vi "Desvio padrão normatizado.vi"(1 "Dados out":T1) -> (0 "Desvios das deformações":dbl[](array[numeric]))   [LabVIEW 2018]
uses:
  Controles/p,q, t, a e b.ctl
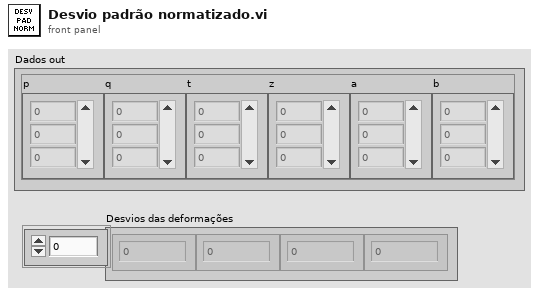
[diagram p1: front panel]
types:
  T1 = typedef "p,q, t, a e b.ctl" = cluster{"p":dbl[], "q":dbl[], "t":dbl[], "z":dbl[], "a":dbl[], "b":dbl[]}
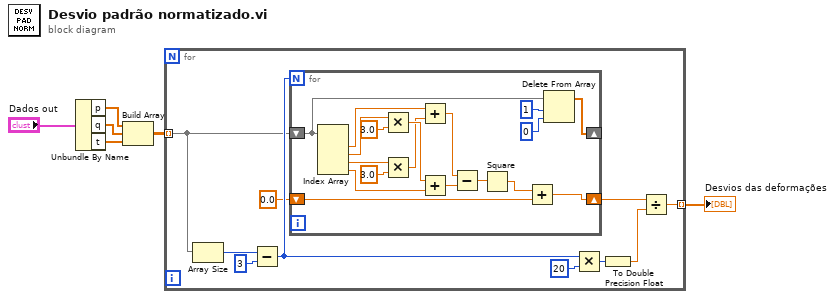
[diagram p0: block diagram]
diagram:
  n1 = Unbundle By Name("Dados out") -> ("p"=w4:dbl[], "q"=w3:dbl[], "t"=w2:dbl[])
  n2 = Build Array(w4, w3, w2) -> (w1:dbl[][])
  n3 = for {
    tunnel: [w10] -> w6 mode=indexing
    tunnel: w1 -> [w9] mode=indexing
    n4 = Array Size(array=w9) -> (size(s)=w16:i32)
    n5 = Subtract(x=w16, y=3) -> (x-y=w13:i32)
    n6 = for {
      N: w13 -> [_]
      shift-right: [w33] -> _
      shift-left: w9 -> [w32]
      shift-right: [w19] -> w11
      shift-left: 0.0 -> [w18]
      n7 = Index Array(array=w32) -> (element #1=w25:dbl, element #2=w31:dbl, element #3=w28:dbl, element #4=w26:dbl)  [unwired: 4 in]
      n8 = Multiply(x=w31, y=3.0) -> (x*y=w27:dbl)
      n9 = Multiply(x=w28, y=3.0) -> (x*y=w24:dbl)
      n10 = Add(x=w25, y=w24) -> (x+y=w23:dbl)
      n11 = Add(x=w27, y=w26) -> (x+y=w22:dbl)
      n12 = Subtract(x=w23, y=w22) -> (x-y=w21:dbl)
      n13 = Square(x=w21) -> (x^2=w20:dbl)
      n14 = Add(x=w20, y=w18) -> (x+y=w19:dbl)
      n15 = Delete From Array(array=w32, length=1, index=0) -> (array with subset deleted=w33:dbl[])  [unwired: 1 out]
    }
    n16 = Multiply(x=w13, y=20) -> (x*y=w8:i32)
    n17 = To Double Precision Float(number=w8) -> (double precision float=w7:dbl)
    n18 = Divide(x=w11, y=w7) -> (x/y=w10:dbl)
  }
  "Desvios das deformações" <- w6
